vi "Ejer 2.vi"() -> ()   [LabVIEW 2020]
panel:
  out "Temperatura":dbl[](graph)
  in  "Stop":bool
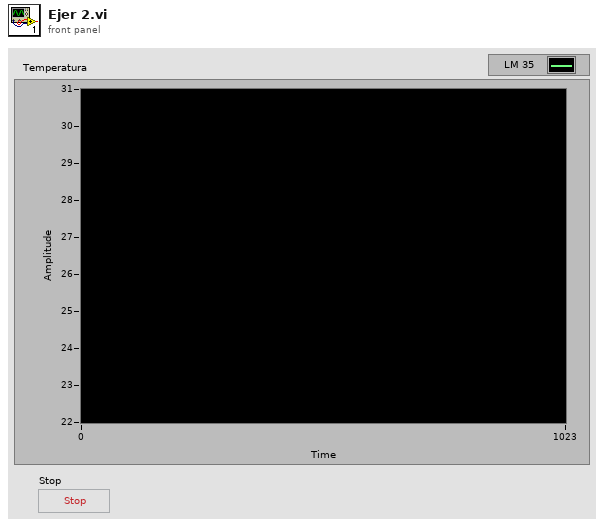
[diagram p1: front panel]
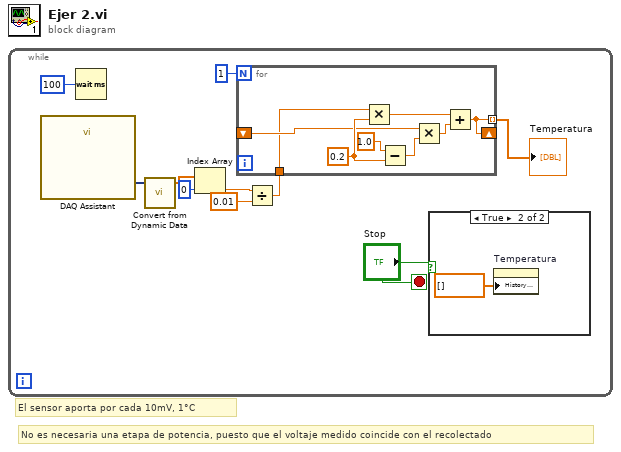
[diagram p0: block diagram]
diagram:
  # "No es necesaria una etapa de potencia, puesto que el voltaje medido coincide con el recolectado"
  # "El sensor aporta por cada 10mV, 1°C"
  n1 = while {
    stop <- "Stop" stop-if-true
    n2 = call "DAQ Assistant"() -> ("data"=w9:dynamicdata)  [unwired: 17 in, 2 out]
    n3 = Wait (ms)(milliseconds to wait=u32 100) -> ()  [unwired: 1 out]
    n4 = call "Convert from Dynamic Data"("Dynamic Data Type"=w9) -> ("Array"=w8:dbl[])  [unwired: 3 in]
    n5 = Index Array(array=w8, index=0) -> (element=w6:dbl)
    n6 = Divide(x=w6, y=0.01) -> (x/y=w2:dbl)
    n7 = for {
      N: 1 -> [_]
      shift-right: [w13] -> _
      shift-left: _ -> [w14]
      tunnel: [w13] -> w3 mode=indexing
      tunnel: w2 -> [w12]
      w16 = 0.2 ("y")
      n8 = Multiply(x=w12, y=w16) -> (x*y=w19:dbl)
      n9 = Subtract(x=1.0, y=w16) -> (x-y=w18:dbl)
      n10 = Multiply(x=w14, y=w18) -> (x*y=w15:dbl)
      n11 = Add(x=w19, y=w15) -> (x+y=w13:dbl)
    }
    "Temperatura" <- w3
    n12 = case shown="True" "Stop" {
      frame False {
      }
      frame True {
        n13 = property on="Temperatura" class="WFChart (strict)"("History Data"=dbl[] []) -> ()  [unwired: 2 in, 2 out]
      }
    }
  }
